vi "Init.vi"(8 "error in (no error)":errorcluster, 11 "UI Actor in":refnum<class "UI Actor.lvclass">) -> (0 "error out":errorcluster, 3 "UI Actor out":refnum<class "UI Actor.lvclass">)   [LabVIEW 2020, in "UI Actor.lvlib" / "UI Actor.lvclass"]
uses:
  UI Actor.lvclass
  C:/Program Files (x86)/National Instruments/LabVIEW 2020/vi.lib/ActorFramework/Actor/Actor.lvclass
  UI Actor.lvclass/UI Actor.ctl
  Monedas MXN/Monedas MXN.lvclass
  Monedas MXN/Monedas MXN.lvclass/Monedas MXN.ctl
  Monedas USD/Monedas USD.lvclass
  Monedas USD/Monedas USD.lvclass/Monedas USD.ctl
  Nestle  Actor/Nestle  Actor.lvclass
  Nestle  Actor/Nestle  Actor.lvclass/Nestle  Actor.ctl
  Coca Actor/Coca Actor.lvclass
  Coca Actor/Coca Actor.lvclass/Coca Actor.ctl
  Read Coins.vi
  Read Sub Panel Coin.vi
  Read Productos.vi
  Read Sub Panel Prod.vi
  <vilib>/ActorFramework/Actor/Actor.lvclass
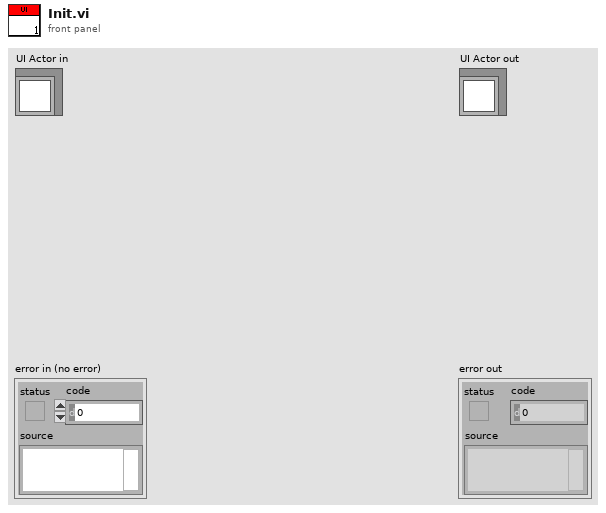
[diagram p1: front panel]
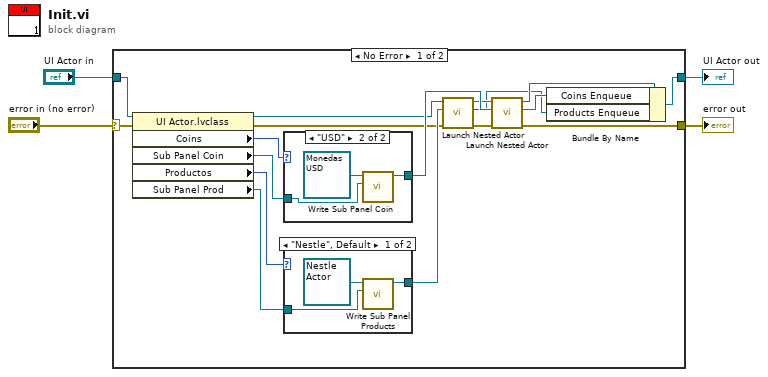
[diagram p0: block diagram]
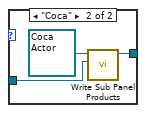
[diagram p2: hidden frame]
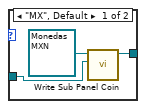
[diagram p3: hidden frame]
diagram:
  n1 = case shown="No Error" "error in (no error)" {
    selector: "error in (no error)" -> [w21 w35]
    tunnel: [w18 w35] -> w3
    tunnel: [w16 w34] -> w1
    tunnel: "UI Actor in" -> [w20 w34]
    frame No Error {
      n2 = property class="UI Actor.lvclass"(reference=w20, error in=w21) -> (reference out=w10:refnum<class "UI Actor.lvclass">, error out=w6:errorcluster, "Coins"=w19:enum16{"MX", "USD"}, "Sub Panel Coin"=w14:refnum<vi>, "Productos"=w12:enum16{"Nestle", "Coca"}, "Sub Panel Prod"=w11:refnum<vi>)
      n3 = case shown="\"USD\"" w19 {
        tunnel: w14 -> [w30 w32]
        tunnel: [w28 w31] -> w13
        frame "MX", Default {
          n4 = call "Write Sub Panel Coin.vi"("Sub Panel Coin"=w30, "Monedas MXN in"=refnum<class "Monedas MXN.lvclass"> refnum ("Monedas MXN.lvlib:Monedas MXN.lvclass")) -> ("Monedas MXN out"=w28:refnum<class "Monedas MXN.lvclass">)  [unwired: 8 in, 1 out]
        }
        frame "USD" {
          n5 = call "Write Sub Panel Coin.vi"("Sub Panel Coin"=w32, "Monedas USD in"=refnum<class "Monedas USD.lvclass"> refnum ("Monedas USD.lvlib:Monedas USD.lvclass")) -> ("Monedas USD out"=w31:refnum<class "Monedas USD.lvclass">)  [unwired: 8 in, 1 out]
        }
      }
      n6 = case shown="\"Nestle\", Default" w12 {
        tunnel: [w23 w26] -> w7
        tunnel: w11 -> [w22 w25]
        frame "Nestle", Default {
          n7 = call "Write Sub Panel Products.vi"("Sub Panel Products"=w22, "Nestle  Actor in"=refnum<class "Nestle  Actor.lvclass"> refnum ("Nestle  Actor.lvlib:Nestle  Actor.lvclass")) -> ("Nestle  Actor out"=w23:refnum<class "Nestle  Actor.lvclass">)  [unwired: 8 in, 1 out]
        }
        frame "Coca" {
          n8 = call "Write Sub Panel Products.vi"("Sub Panel Products"=w25, "Coca Actor in"=refnum<class "Coca Actor.lvclass"> refnum ("Coca Actor.lvlib:Coca Actor.lvclass")) -> ("Coca Actor out"=w26:refnum<class "Coca Actor.lvclass">)  [unwired: 8 in, 1 out]
        }
      }
      n9 = call <vilib>:"Launch Nested Actor.vi"("error in (no error)"=w6, "Nested Actor"=w7, "Caller Actor in"=w10) -> ("error out"=w5:errorcluster, "Nested Actor's Enqueuer"=w8:refnum<class "Message Enqueuer.lvclass">, "Caller Actor out"=w9:refnum<class "UI Actor.lvclass">)  [unwired: 6 in]
      n10 = call <vilib>:"Launch Nested Actor.vi"("error in (no error)"=w5, "Nested Actor"=w13, "Caller Actor in"=w9) -> ("error out"=w18:errorcluster, "Nested Actor's Enqueuer"=w15:refnum<class "Message Enqueuer.lvclass">, "Caller Actor out"=w17:refnum<class "UI Actor.lvclass">)  [unwired: 6 in]
      n11 = Bundle By Name(cluster=w17, "Coins Enqueue"=w15, "Products Enqueue"=w8) -> (w16:refnum<class "UI Actor.lvclass">)
    }
    frame Error {
    }
  }
  "error out" <- w3
  "UI Actor out" <- w1
